vi "LED_flag.vi"() -> ()   [LabVIEW 2020]
panel:
  in  "stop":bool
  out "x/y":dbl
  in  "x":dbl
  out "Error! Divided by Zero":bool
  in  "y":dbl
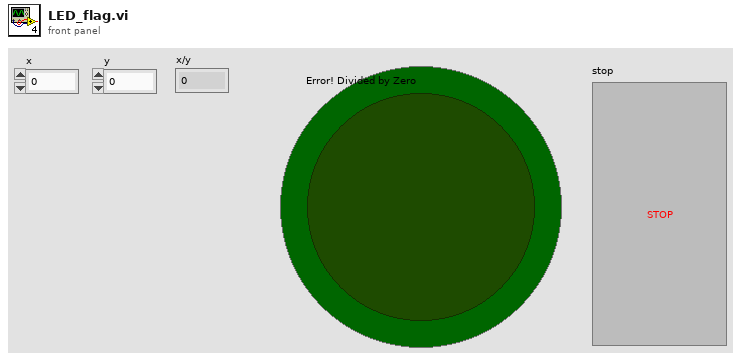
[diagram p1: front panel]
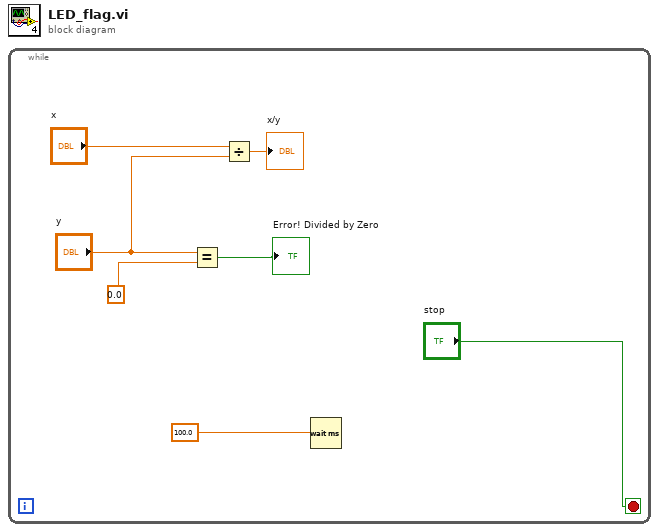
[diagram p0: block diagram]
diagram:
  n1 = while {
    stop <- "stop" stop-if-true
    n2 = Equal?(x="y", y=0.0) -> (x = y?=→"Error! Divided by Zero":bool)
    n3 = Divide(x="x", y="y") -> (x/y=→"x/y":dbl)
    n4 = Wait (ms)(milliseconds to wait=100.0) -> ()  [unwired: 1 out]
  }
